vi "Not An Agent Public Key.vi"(1 "agent public key":T1) -> (0 "Not a Agent Public Key?":bool)   [LabVIEW 2013, in "libssh2.lvlib"]
doc: "Returns TRUE if <B>agent public key</B> is not an agent public key. Otherwise, FALSE."
uses:
  libssh2.lvlib
  Agent Public Key Refnum.ctl
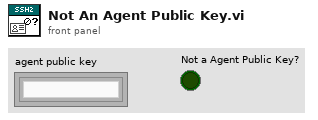
[diagram p1: front panel]
types:
  T1 = typedef "libssh2.lvlib/Agent Public Key Refnum.ctl" = refnum<k1>
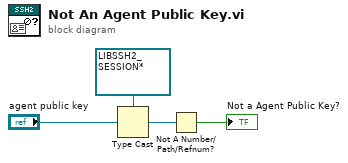
[diagram p0: block diagram]
diagram:
  n1 = Type Cast(type=refnum<data-value> refnum ("data value reference"), x="agent public key") -> (*(type *) &x=w2:refnum<data-value>)
  n2 = Not A Number/Path/Refnum?(number/path/refnum=w2) -> (NaN/Path/Refnum?=→"Not a Agent Public Key?":bool)
